vi "Read Error.vi"(8 "error in (no error)":errorcluster, 11 "Data Msg in":refnum<class "Data Msg.lvclass">) -> (0 "error out":errorcluster, 2 "Error?":bool, 3 "Data Msg out":refnum<class "Data Msg.lvclass">)   [LabVIEW 2014, in "Data Msg.lvclass"]
uses:
  Data Msg.lvclass
  Data Msg.lvclass/Data Msg.ctl
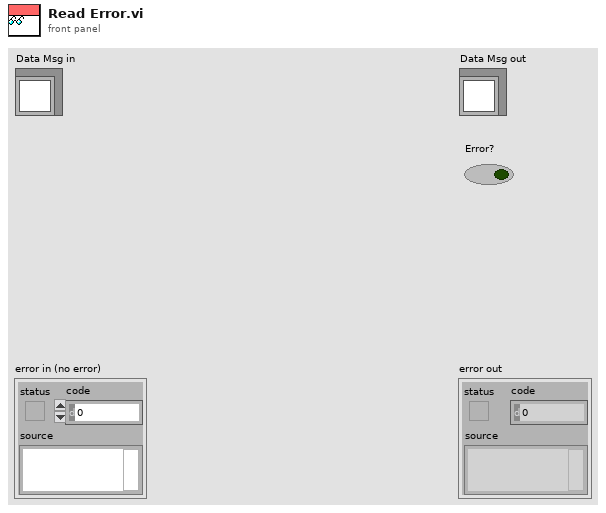
[diagram p1: front panel]
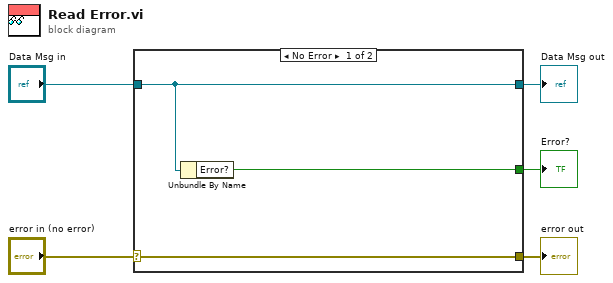
[diagram p0: block diagram]
diagram:
  n1 = case shown="No Error" "error in (no error)" {
    selector: "error in (no error)" -> [w8 w9]
    tunnel: [w8 w9] -> w4
    tunnel: [w7 w10] -> w2
    tunnel: "Data Msg in" -> [w7 w10]
    tunnel: [w6 _] -> w1
    frame No Error {
      n2 = Unbundle By Name(w7) -> ("Error?"=w6:bool)
    }
    frame Error {
    }
  }
  "error out" <- w4
  "Data Msg out" <- w2
  "Error?" <- w1
